vi "tt20panel_set_chart_properties.vi"(8 "error in (no error)":errorcluster, 11 "panel.lvclass":refnum<class "panel.lvclass">) -> (0 "error in (no error) 2":errorcluster, 3 "panel out":refnum<class "panel.lvclass">)   [LabVIEW 2015, in "tt20panel.lvclass"]
uses:
  tt20panel.lvclass
  UI/panel_class/panel.lvclass
  UI/panel_class/panel.lvclass/panel.ctl
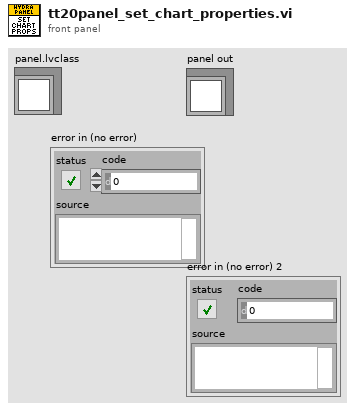
[diagram p1: front panel]
types:
  T1 = typedef "ui_plot_references.ctl" = cluster{"plots":refnum<vi>, "chart":refnum<vi>, "graph":refnum<vi>, "map":refnum<vi>, "XY Graph":refnum<vi>}
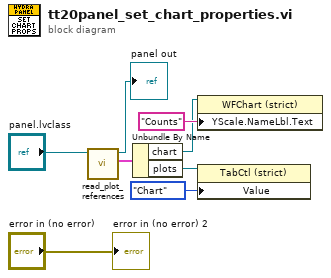
[diagram p0: block diagram]
diagram:
  n1 = call "read_plot_references.vi"("panel in"="panel.lvclass") -> ("plot_references"=w5:T1, "panel out"=→"panel out":refnum<class "panel.lvclass">)  [unwired: 8 in, 1 out]
  n2 = Unbundle By Name(w5) -> ("chart"=w4:refnum<vi>, "plots"=w7:refnum<vi>)
  n3 = property class="WFChart (strict)"(reference=w4, "YScale.NameLbl.Text"="Counts" ("Y Scale.Name Label.Text")) -> ()  [unwired: 1 in, 2 out]
  n4 = property class="TabCtl (strict)"(reference=w7, "Value"=enum32{"Chart", "Graph", "Map", "XY Graph"}."Chart") -> ()  [unwired: 1 in, 2 out]
  "error in (no error) 2" <- "error in (no error)"
